vi "CalcHypotenuse.vi"(4 "b":dbl, 5 "a":dbl) -> (1 "hypotenuse":dbl)   [LabVIEW 2017]
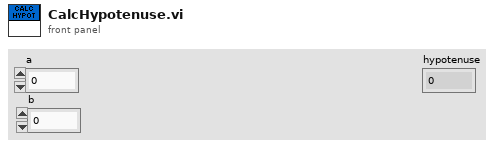
[diagram p1: front panel]
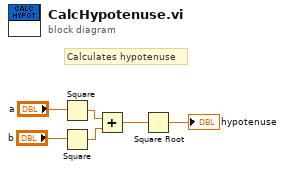
[diagram p0: block diagram]
diagram:
  # "Calculates hypotenuse"
  n1 = Square(x="a") -> (x^2=w6:dbl)
  n2 = Square(x="b") -> (x^2=w5:dbl)
  n3 = Add(x=w6, y=w5) -> (x+y=w4:dbl)
  n4 = Square Root(x=w4) -> (sqrt(x)=→"hypotenuse":dbl)
